vi "add open sr830(SubVI).vi"() -> (1 "ok or cancel":bool, 2 "open":string)   [LabVIEW 2019, in "Add Seq.lvlib"]
uses:
  Add Seq.lvlib
panel:
  in  "cancel":bool
  in  "ok":bool
  in  "SR830 VISA 4":bool
  in  "SR830 VISA 3":bool
  in  "SR830 VISA 2":bool
  in  "SR830 VISA 1":bool
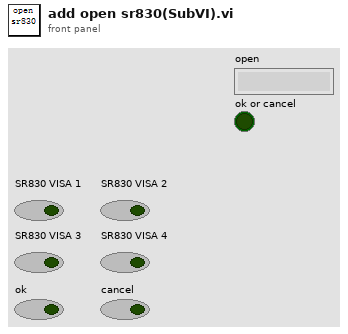
[diagram p1: front panel]
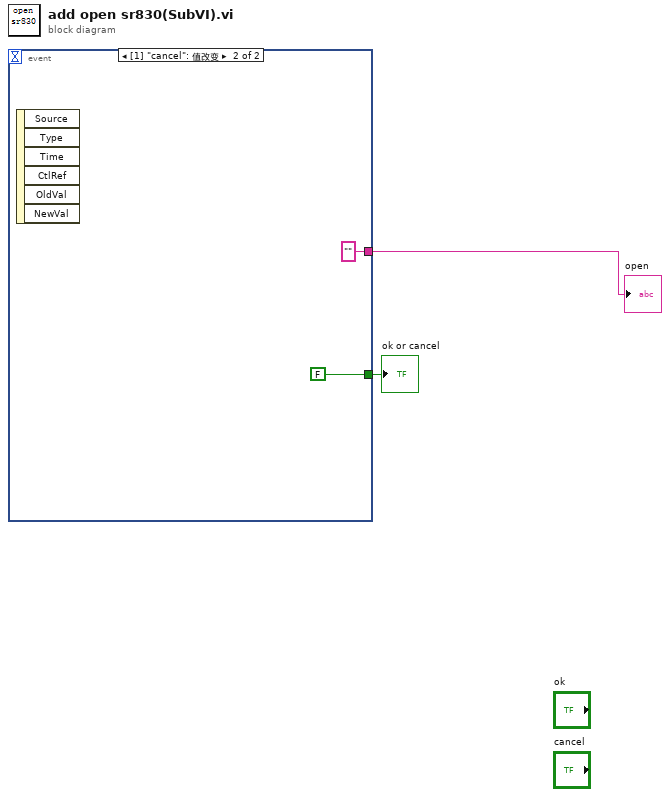
[diagram p0: block diagram]
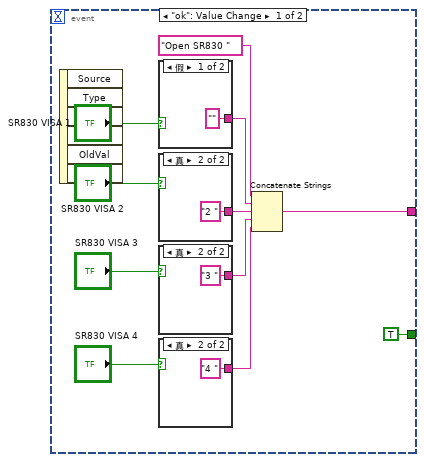
[diagram p2: hidden frame]
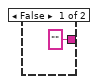
[diagram p3: hidden frame]
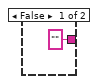
[diagram p4: hidden frame]
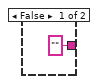
[diagram p5: hidden frame]
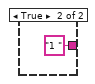
[diagram p6: hidden frame]
diagram:
  n1 = event shown="[1] \"cancel\": 值改变" {
    selector: _ -> [_ _]
    dyn-events: _ -> [_ _]
    timeout: _ -> [_ _]
    tunnel: [w4 ""] -> w2
    tunnel: [TRUE FALSE] -> w1
    event "ok": Value Change {
      n2 = event-data() -> ()  [unwired: 1 in, 6 out]
      n3 = case shown="假" "SR830 VISA 1" {
        tunnel: ["" "1 "] -> w11
        frame False {
        }
        frame True {
        }
      }
      n4 = case shown="真" "SR830 VISA 2" {
        tunnel: ["" "2 "] -> w7
        frame False {
        }
        frame True {
        }
      }
      n5 = case shown="真" "SR830 VISA 3" {
        tunnel: ["" "3 "] -> w6
        frame False {
        }
        frame True {
        }
      }
      n6 = case shown="真" "SR830 VISA 4" {
        tunnel: ["" "4 "] -> w5
        frame False {
        }
        frame True {
        }
      }
      n7 = Concatenate Strings("Open SR830 ", w11, w7, w6, w5) -> (w4:string)
    }
    event "cancel": Value Change {
      n8 = event-data() -> ()  [unwired: 1 in, 6 out]
    }
  }
  "open" <- w2
  "ok or cancel" <- w1
